vi "SyncClock.vi"(8 "error in (no error)":errorcluster caption="错误输入（无错误）", 9 "clcChoice":dbl, 10 "syncChoice":dbl, 11 "Path":path) -> (0 "error out":errorcluster caption="错误输出", 3 "syncClock":u8)   [LabVIEW 2015]
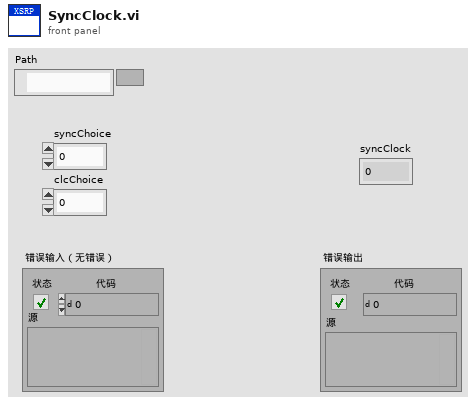
[diagram p1: front panel]
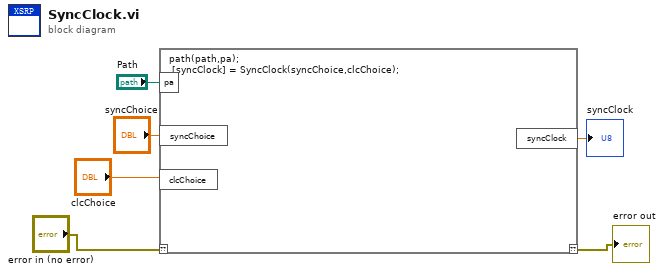
[diagram p0: block diagram]
diagram:
  n1 = script code="path(path,pa);\n [syncClock] = SyncClock(syncChoice,clcChoice);"("??"="error in (no error)", "pa"="Path", "syncChoice"="syncChoice", "clcChoice"="clcChoice") -> ("??"=→"error out":errorcluster, "syncClock"=→"syncClock":dbl)
